vi "Read t0.vi"(8 "error in (no error)":errorcluster, 11 "Const_WFM in":refnum<class "Const_WFM_1D.lvclass">) -> (0 "error out":errorcluster, 2 "t0":timestamp[](array[timestamp]), 3 "Const_WFM out":refnum<class "Const_WFM_1D.lvclass">)   [LabVIEW 2021, in "Const_WFM_1D.lvclass"]
uses:
  Const_WFM_1D.lvclass
  Const_WFM_1D.lvclass/Const_WFM_1D.ctl
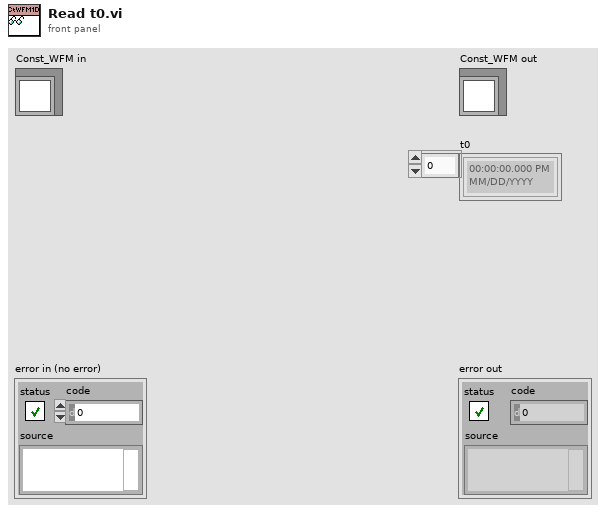
[diagram p1: front panel]
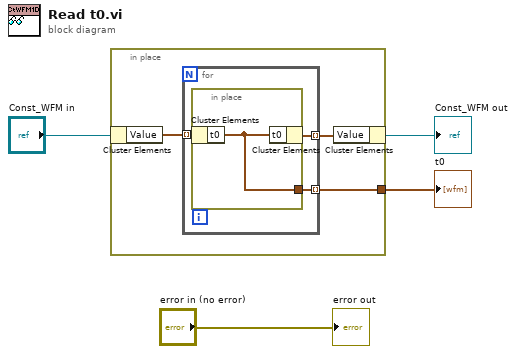
[diagram p0: block diagram]
diagram:
  n1 = in-place {
    in-place-border: [w5] -> w1
    n2 = in-place-cluster #1("Const_WFM in") -> ("Value"=w7:waveform(dbl)[])
    n3 = for {
      tunnel: w7 -> [w10] mode=indexing
      tunnel: [w9] -> w6 mode=indexing
      tunnel: [w8] -> w5 mode=indexing
      n4 = in-place {
        in-place-border: [w11] -> w8
        n5 = in-place-cluster #2(w10) -> ("t0"=w11:timestamp)
        n6 = in-place-cluster #2("t0"=w11) -> (w9:waveform(dbl))
      }
    }
    n7 = in-place-cluster #1("Value"=w6) -> (→"Const_WFM out":refnum<class "Const_WFM_1D.lvclass">)
  }
  "t0" <- w1
  "error out" <- "error in (no error)"
